vi "Rangos.vi"() -> ()   [LabVIEW 2011]
panel:
  out "Maximo":dbl
  out "Minimo":dbl
  in  "Boolean":bool
  out "Rango de 151-220":bool
  out "Rango de 101-150":bool
  out "Rango de 1-100":bool
  out "Rango de 151-220":dbl
  out "Rango de 101-150":dbl
  out "Rango de 1-100":dbl
  out "Gauge":dbl(knob) scale=0.0..220.0
  # "Se tiene que contar cuantas veces la velocidad genera en caada una de los\nrangos y se enciende el led que corresponde a cada uno de los rangos\nhacerlo hasta pagar el auto"
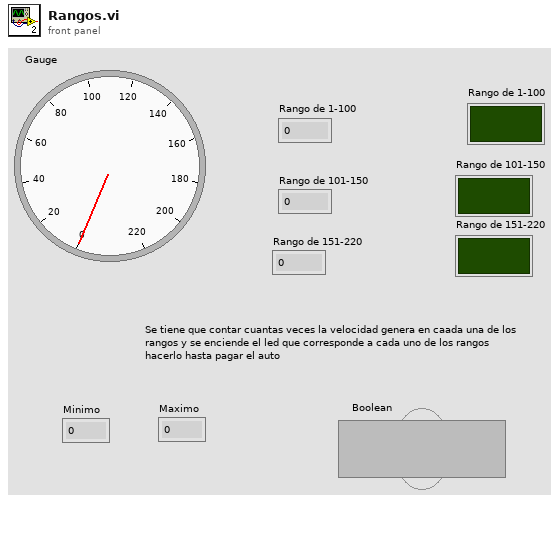
[diagram p1: front panel]
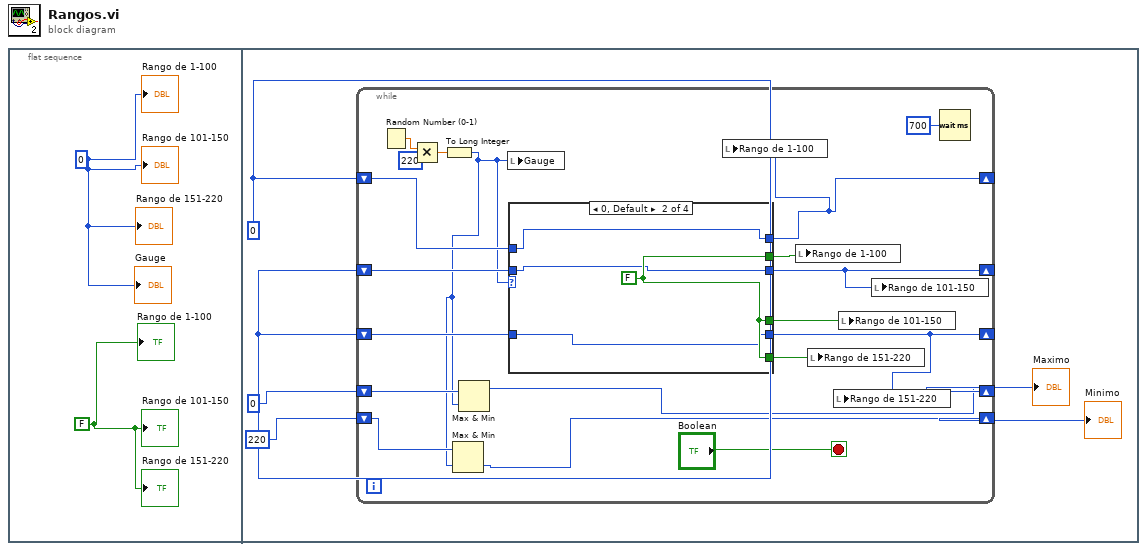
[diagram p0: block diagram]
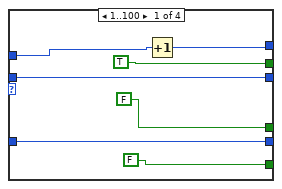
[diagram p2: hidden frame]
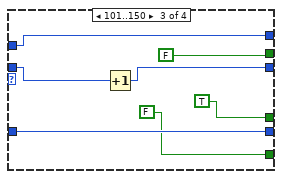
[diagram p3: hidden frame]
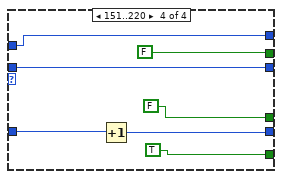
[diagram p4: hidden frame]
diagram:
  n1 = flat-sequence {
    frame #0 {
      w2 = 0
      w1 = FALSE
      "Gauge" <- w2
      "Rango de 1-100" <- w2
      "Rango de 101-150" <- w2
      "Rango de 151-220" <- w2
      "Rango de 1-100" <- w1
      "Rango de 101-150" <- w1
      "Rango de 151-220" <- w1
    }
    frame #1 {
      w6 = 0
      n2 = while {
        shift-right: [w20] -> _
        shift-left: w6 -> [w23]
        shift-right: [w16] -> _
        shift-left: w6 -> [w22]
        shift-right: [w15] -> _
        shift-left: w6 -> [w21]
        shift-right: [w8] -> w5
        shift-left: 0 -> [w12]
        shift-right: [w9] -> w4
        shift-left: 220 -> [w11]
        stop <- "Boolean" stop-if-true
        n3 = Random Number (0-1)() -> (number: 0 to 1=w26:dbl)
        n4 = Multiply(x=w26, y=220) -> (x*y=w24:dbl)
        n5 = To Long Integer(number=w24) -> (32bit integer=w10:i32)
        n6 = Max & Min(x=w11, y=w10) -> (min(x,y)=w9:i32)  [unwired: 1 out]
        n7 = Max & Min(x=w12, y=w10) -> (max(x,y)=w8:i32)  [unwired: 1 out]
        n8 = local write "Gauge"(w10) -> ()
        n9 = case shown="0, Default" w10 {
          tunnel: [w30 w36 w38 w51] -> w20
          tunnel: w23 -> [w31 w36 w38 w51]
          tunnel: [w33 w35 w43 w50] -> w16
          tunnel: w22 -> [w33 w35 w44 w50]
          tunnel: [w32 w34 w42 w48] -> w15
          tunnel: w21 -> [w32 w34 w42 w49]
          tunnel: [TRUE w37 FALSE FALSE] -> w19
          tunnel: [FALSE w37 TRUE FALSE] -> w18
          tunnel: [FALSE w37 FALSE TRUE] -> w17
          frame 1..100 {
            n10 = Increment(x=w31) -> (x+1=w30:i32)
          }
          frame 0, Default {
            w37 = FALSE
          }
          frame 101..150 {
            n11 = Increment(x=w44) -> (x+1=w43:i32)
          }
          frame 151..220 {
            n12 = Increment(x=w49) -> (x+1=w48:i32)
          }
        }
        n13 = local write "Rango de 1-100"(w20) -> ()
        n14 = local write "Rango de 1-100"(w19) -> ()
        n15 = local write "Rango de 151-220"(w17) -> ()
        n16 = local write "Rango de 151-220"(w15) -> ()
        n17 = local write "Rango de 101-150"(w18) -> ()
        n18 = local write "Rango de 101-150"(w16) -> ()
        n19 = Wait (ms)(milliseconds to wait=u32 700) -> ()  [unwired: 1 out]
      }
      "Maximo" <- w5
      "Minimo" <- w4
    }
  }
